vi "StreamEngine.Main.Stream.BusData.Process.vi"(8 "error in (no error)":errorcluster, 9 "Host Parameters":T1, 10 "Init?":bool, 11 "frame":T5[](array[typedef])) -> (0 "error out":errorcluster, 2 "Table Update":bool, 3 "Table":string[][](array[string]))   [LabVIEW 2025, in "XNET Bus Monitor Client.lvlib"]
uses:
  XNET Bus Monitor Client.lvlib
  xnet_can_bus_monitor_api_client/RPC Messages/ni_xnet_can_bm_api_Frame.ctl
  Types/StreamEngine.Parameters.ctl
  xnet_can_bus_monitor_api_client/RPC Messages/ni_xnet_can_bm_api_FilterInfo.ctl
  xnet_can_bus_monitor_api_client/RPC Messages/ni_xnet_can_bm_api_DirectionFilter.ctl
  xnet_can_bus_monitor_api_client/RPC Messages/ni_xnet_can_bm_api_FrameFilter.ctl
  <vilib>/dlg_ctls.llb/Space Constant.vi
  <vilib>/Utility/error.llb/Trim Whitespace.vi
  Convert.TimeToUTCString.vi
  <vilib>/Utility/error.llb/Trim Whitespace One-Sided.vi
  <userlib>/_OpenG.lib/array/array.llb/Sort 2D Array (String)__ogtk.vi
  <userlib>/_OpenG.lib/array/array.llb/openg_array.lvlib
  xnet_can_bus_monitor_api_client/xnet_can_bus_monitor_api_client.lvlib
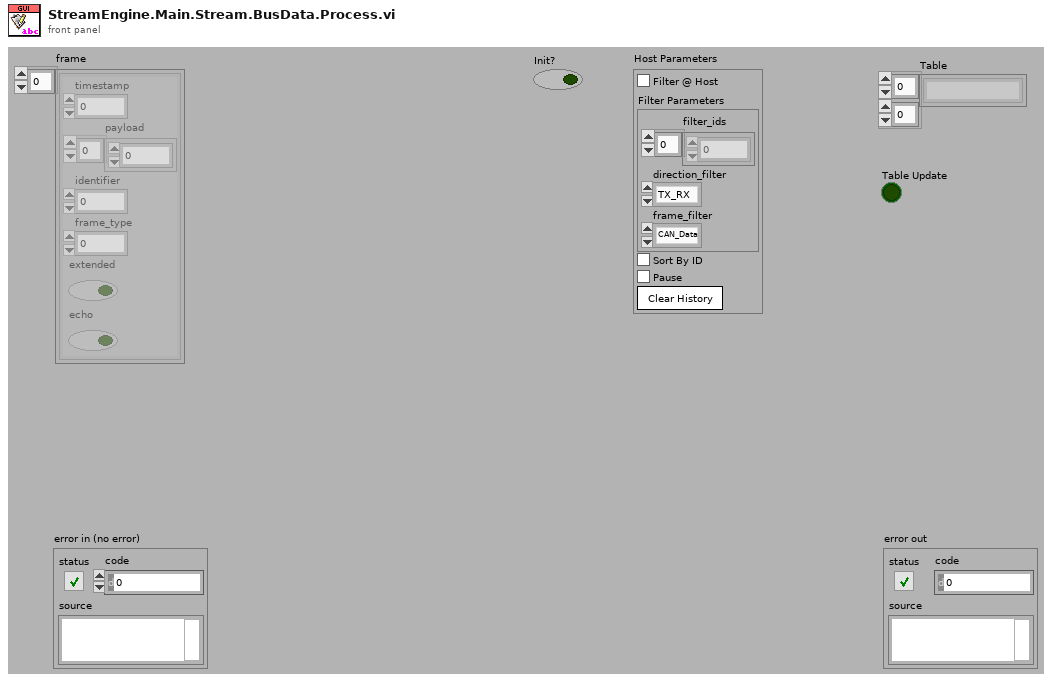
[diagram p1: front panel]
types:
  T1 = typedef "XNET Bus Monitor Client.lvlib/StreamEngine.Parameters.ctl" = cluster{"Host Filter":bool, "Filter Parameters":T2, "Sort By ID":bool, "Pause":bool, "Clear History":bool}
  T2 = typedef "xnet_can_bus_monitor_api_client.lvlib/ni_xnet_can_bm_api_FilterInfo.ctl" = cluster{"filter_ids":u32[], "direction_filter":T3, "frame_filter":T4}
  T3 = typedef "xnet_can_bus_monitor_api_client.lvlib/ni_xnet_can_bm_api_DirectionFilter.ctl" = enum32{"TX_RX", "RX", "TX"}
  T4 = typedef "xnet_can_bus_monitor_api_client.lvlib/ni_xnet_can_bm_api_FrameFilter.ctl" = enum32{"CAN_Data", "CAN_Remote", "CAN_Bus_Error", "CAN_2_Data", "CAN_FD_Data", "CAN_FD_BRS_Data", "J1939_Data", "Delay", "Log_Trigger", "Start_Trigger", "All"}
  T5 = typedef "xnet_can_bus_monitor_api_client.lvlib/ni_xnet_can_bm_api_Frame.ctl" = cluster{"timestamp":dbl, "payload":u8[], "identifier":u32, "frame_type":u32, "extended":bool, "echo":bool}
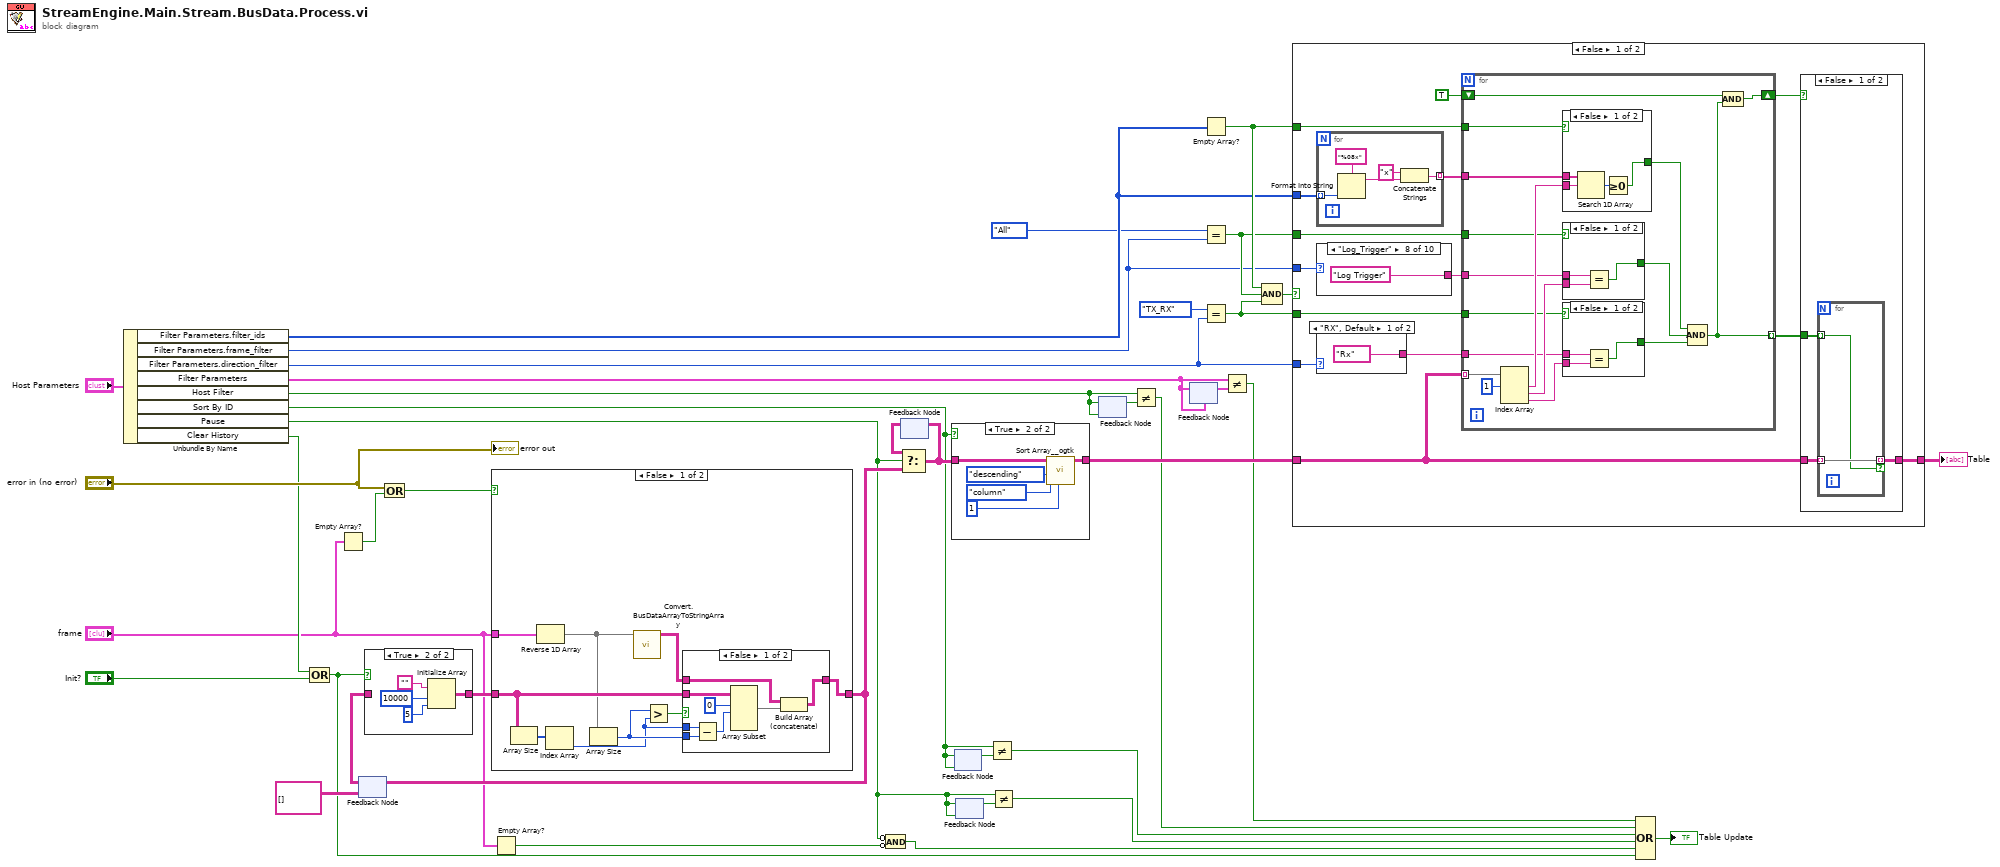
[diagram p0: block diagram]
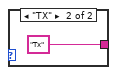
[diagram p4: hidden frame]
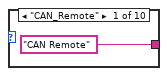
[diagram p5: hidden frame]
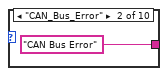
[diagram p6: hidden frame]
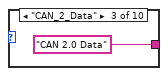
[diagram p7: hidden frame]
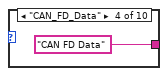
[diagram p8: hidden frame]
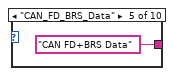
[diagram p9: hidden frame]
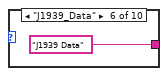
[diagram p10: hidden frame]
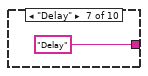
[diagram p11: hidden frame]
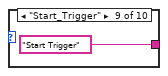
[diagram p12: hidden frame]
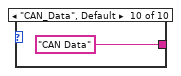
[diagram p13: hidden frame]
diagram:
  n1 = Unbundle By Name("Host Parameters") -> ("Filter Parameters.filter_ids"=w21:u32[], "Filter Parameters.frame_filter"=w20:T4, "Filter Parameters.direction_filter"=w19:T3, "Filter Parameters"=w13:T2, "Host Filter"=w10:bool, "Sort By ID"=w5:bool, "Pause"=w2:bool, "Clear History"=w30:bool)
  n2 = Compound Arithmetic op=OR(w30, "Init?") -> (w28:bool)
  n3 = Empty Array?(array="frame") -> (empty?=w15:bool)
  n4 = feedback #1(string[][] [] ("Sorted Array out")) -> (w39:string[][])
  n5 = case shown="True" w28 {
    tunnel: [w41 w43] -> w40
    tunnel: w39 -> [w41 _]
    frame False {
    }
    frame True {
      n6 = Initialize Array("", 10000 ("dimension size"), 5 ("Dimension Size")) -> (w43:string[][])
    }
  }
  n7 = Compound Arithmetic op=OR("error in (no error)", w15) -> (w34:bool)
  n8 = case shown="False" w34 {
    tunnel: "frame" -> [w46 _]
    tunnel: w40 -> [w50 w64]
    tunnel: [w51 w64] -> w37
    frame False {
      n9 = Array Size(array=w50) -> (size(s)=w49:i32[])
      n10 = Reverse 1D Array(array=w46) -> (reversed array=w47:T5[])
      n11 = Index Array(array=w49) -> (element=w48:i32)  [unwired: 1 in]
      n12 = Array Size(array=w47) -> (size(s)=w52:i32)
      n13 = call "Convert.BusDataArrayToStringArray.vi"("frame"=w47) -> ("Array out"=w53:string[][])  [unwired: 10 in]
      n14 = Greater?(x=w52, y=w48) -> (0:w54:bool)
      n15 = case shown="False" w54 {
        tunnel: w53 -> [w56 w63]
        tunnel: w48 -> [w62 _]
        tunnel: [w55 w63] -> w51
        tunnel: w50 -> [w60 _]
        tunnel: w52 -> [w61 _]
        frame False {
          n16 = Subtract(x=w62, y=w61) -> (x-y=w58:i32)
          n17 = Array Subset(array=w60, index (row)=0 ("index"), length (row)=w58) -> (w57:string[][])  [unwired: 2 in]
          n18 = Build Array (concatenate)(w56, w57) -> (w55:string[][])
        }
        frame True {
        }
      }
    }
    frame True {
    }
  }
  n19 = feedback-in #1(w37) -> ()
  n20 = Empty Array?(array="frame") -> (empty?=w7:bool)
  n21 = Compound Arithmetic op=AND(invert w2, invert w7) -> (w8:bool)
  n22 = feedback #2() -> (w36:string[][])  [unwired: 1 in]
  n23 = Select(t=w36, s=w2, f=w37) -> (s? t:f=w33:string[][])
  n24 = feedback-in #2(w33) -> ()
  n25 = case shown="True" w5 {
    tunnel: w33 -> [w65 w70]
    tunnel: [w65 w69] -> w27
    frame False {
    }
    frame True {
      n26 = call-poly <userlib>:"Sort Array__ogtk.vi"("Column/Row to Sort By"=u32 1, "Sort By in"=enum16{"row", "column"}."column", "Order"=enum16{"ascending", "descending"}."descending", "Array in"=w70) -> ("Sorted Array out"=w69:string[][])  [unwired: 4 in, 3 out]
    }
  }
  n27 = feedback #3(w5) -> (w6:bool)
  n28 = feedback-in #3(w5) -> ()
  n29 = feedback #4(w2) -> (w3:bool)
  n30 = feedback-in #4(w2) -> ()
  n31 = Not Equal?(x=w5, y=w6) -> (x != y?=w4:bool)
  n32 = Not Equal?(x=w2, y=w3) -> (x != y?=w1:bool)
  n33 = feedback #5(w10) -> (w11:bool)
  n34 = feedback-in #5(w10) -> ()
  n35 = Not Equal?(x=w10, y=w11) -> (x != y?=w9:bool)
  n36 = feedback-in #6(w13) -> ()
  n37 = feedback #6(w13) -> (w14:T2)
  n38 = Empty Array?(array=w21) -> (empty?=w24:bool)
  n39 = Equal?(x=ni_xnet_can_bm_api_FrameFilter."All" ("Filter Parameters.frame_filter"), y=w20) -> (x = y?=w22:bool)
  n40 = Equal?(x=ni_xnet_can_bm_api_DirectionFilter."TX_RX" ("direction_filter"), y=w19) -> (x = y?=w23:bool)
  n41 = Not Equal?(x=w13, y=w14) -> (x != y?=w12:bool)
  n42 = Compound Arithmetic op=AND(w24, w22, w23) -> (w26:bool)
  n43 = case shown="False" w26 {
    tunnel: w27 -> [w78 w138]
    tunnel: w22 -> [w84 _]
    tunnel: w23 -> [w83 _]
    tunnel: [w77 w138] -> w25
    tunnel: w24 -> [w82 _]
    tunnel: w21 -> [w76 _]
    tunnel: w20 -> [w74 _]
    tunnel: w19 -> [w72 _]
    frame False {
      n44 = for {
        tunnel: w76 -> [w98] mode=indexing
        tunnel: [w97] -> w75 mode=indexing
        n45 = Format Into String(format string="%08x", w98) -> (resulting string=w100:string)  [unwired: 2 in, 1 out]
        n46 = Concatenate Strings("x" ("string"), w100) -> (w97:string)
      }
      n47 = case shown="\"Log_Trigger\"" w74 {
        tunnel: ["CAN Remote" "CAN Bus Error" "CAN 2.0 Data" "CAN FD Data" "CAN FD+BRS Data" "J1939 Data" "Delay" "Log Trigger" "Start Trigger" "CAN Data"] -> w73
        frame "CAN_Remote" {
        }
        frame "CAN_Bus_Error" {
        }
        frame "CAN_2_Data" {
        }
        frame "CAN_FD_Data" {
        }
        frame "CAN_FD_BRS_Data" {
        }
        frame "J1939_Data" {
        }
        frame "Delay" {
        }
        frame "Log_Trigger" {
        }
        frame "Start_Trigger" {
        }
        frame "CAN_Data", Default {
        }
      }
      n48 = case shown="\"RX\", Default" w72 {
        tunnel: ["Rx" "Tx"] -> w71
        frame "RX", Default {
        }
        frame "TX" {
        }
      }
      n49 = for {
        tunnel: w78 -> [w122] mode=indexing
        tunnel: w84 -> [w109]
        tunnel: w73 -> [w110]
        tunnel: w71 -> [w111]
        tunnel: w83 -> [w112]
        tunnel: w75 -> [w123]
        tunnel: w82 -> [w124]
        tunnel: [w115] -> w80 mode=indexing
        shift-right: [w114] -> w79
        shift-left: TRUE -> [w116]
        n50 = Index Array(array=w122, index #1=1 ("index")) -> (element #1=w121:string, element #2=w120:string, element #3=w108:string)  [unwired: 2 in]
        n51 = case shown="False" w124 {
          selector: w124 -> [_ w129]
          tunnel: w123 -> [w128 _]
          tunnel: w121 -> [w127 _]
          tunnel: [w125 w129] -> w119
          frame False {
            n52 = Search 1D Array(1D array=w128, element=w127) -> (index of element=w126:i32)  [unwired: 1 in]
            n53 = Greater Or Equal To 0?(x=w126) -> (x >= 0?=w125:bool)
          }
          frame True {
          }
        }
        n54 = case shown="False" w109 {
          selector: w109 -> [_ w133]
          tunnel: w110 -> [w132 _]
          tunnel: [w131 w133] -> w118
          tunnel: w120 -> [w130 _]
          frame False {
            n55 = Equal?(x=w132, y=w130) -> (x = y?=w131:bool)
          }
          frame True {
          }
        }
        n56 = case shown="False" w112 {
          selector: w112 -> [_ w137]
          tunnel: w111 -> [w136 _]
          tunnel: [w135 w137] -> w117
          tunnel: w108 -> [w134 _]
          frame False {
            n57 = Equal?(x=w136, y=w134) -> (x = y?=w135:bool)
          }
          frame True {
          }
        }
        n58 = Compound Arithmetic op=AND(w119, w118, w117) -> (w115:bool)
        n59 = Compound Arithmetic op=AND(w116, w115) -> (w114:bool)
      }
      n60 = case shown="False" w79 {
        tunnel: w78 -> [w102 w107]
        tunnel: [w103 w107] -> w77
        tunnel: w80 -> [w104 _]
        frame False {
          n61 = for {
            tunnel: w104 -> [w105] mode=indexing
            tunnel: [w106] -> w103 mode=indexing if=w105
            tunnel: w102 -> [w106] mode=indexing
          }
        }
        frame True {
        }
      }
    }
    frame True {
    }
  }
  "Table" <- w25
  n62 = Compound Arithmetic op=OR(w12, w9, w4, w1, w8, w28) -> (→"Table Update":bool)
  "error out" <- "error in (no error)"
